vi "API String - List Boolean Strings.vi"(8 "Error in":errorcluster caption="Error in (no error)") -> (0 "Error out":errorcluster, 2 "False Boolean Strings":string[](array[string]), 3 "True Boolean Strings":string[](array[string]))   [LabVIEW 2017, in "API String Arguments Support.lvlib"]
uses:
  API String Arguments Support.lvlib
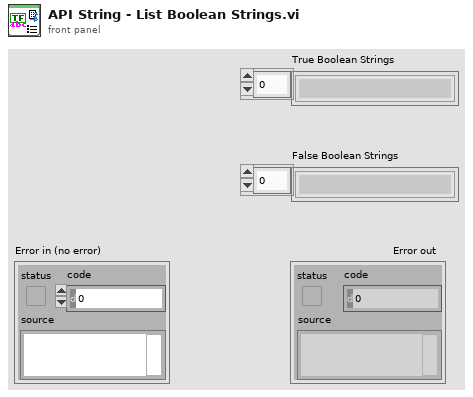
[diagram p1: front panel]
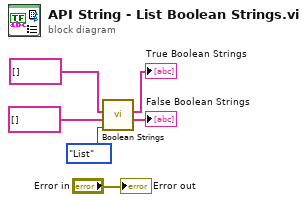
[diagram p0: block diagram]
diagram:
  n1 = call "Boolean Strings.vi"("Enum"=enum16{"List", "Add", "Remove"}."List", "Customer False Boolean Strings"=string[] [], "Customer True Boolean Strings"=string[] []) -> ("False Boolean Strings"=→"False Boolean Strings":string[], "True Boolean Strings"=→"True Boolean Strings":string[])  [unwired: 5 in, 2 out]
  "Error out" <- "Error in"
